vi "VsEP-Append Data.vi"(0 "path":path, 7 "Analysis":T2, 9 "Notes":string, 11 "error in (no error)":errorcluster) -> (15 "error out":errorcluster)   [LabVIEW 2020]
uses:
  Typedefs/VsEP-Analysis State.ctl
panel:
  in  "Data":T1
  out "path out":path
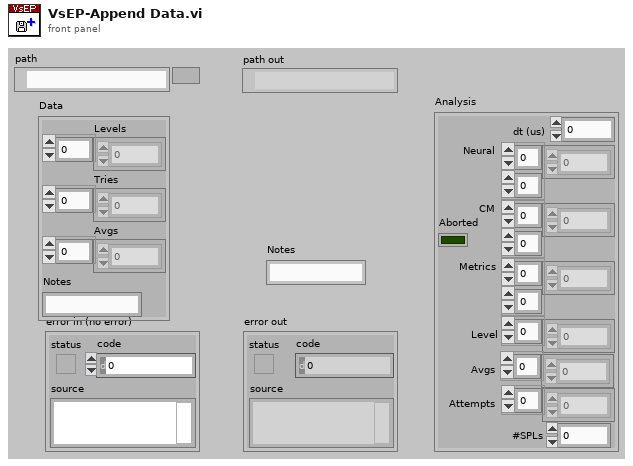
[diagram p1: front panel]
types:
  T1 = cluster{"Levels":dbl[], "Tries":i32[], "Avgs":i32[], "Notes":string}
  T2 = typedef "VsEP-Analysis State.ctl" = cluster{"dt (us)":dbl, "Neural":dbl[][], "CM":dbl[][], "Metrics":dbl[][], "Level":dbl[], "Avgs":i32[], "Attempts":i32[], "Aborted":bool, "#SPLs":i32}
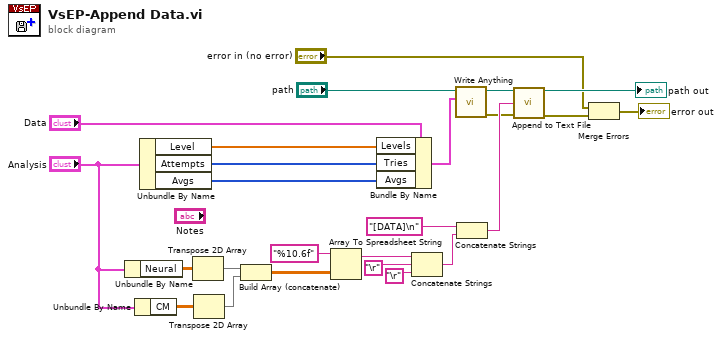
[diagram p0: block diagram]
diagram:
  n1 = Unbundle By Name("Analysis") -> ("Neural"=w15:dbl[][])
  n2 = Unbundle By Name("Analysis") -> ("CM"=w13:dbl[][])
  n3 = Unbundle By Name("Analysis") -> ("Level"=w9:dbl[], "Attempts"=w8:i32[], "Avgs"=w7:i32[])
  n4 = Transpose 2D Array(2D array=w15) -> (transposed array=w18:dbl[][])
  n5 = Transpose 2D Array(2D array=w13) -> (transposed array=w17:dbl[][])
  n6 = Build Array (concatenate)(w18, w17) -> (w16:dbl[][])
  n7 = Array To Spreadsheet String(array=w16, 3:"%10.6f") -> (spreadsheet string=w22:string)  [unwired: 1 in]
  n8 = Bundle By Name(cluster="Data", "Levels"=w9, "Tries"=w8, "Avgs"=w7) -> (w3:T1)
  n9 = Concatenate Strings(w22, "\r", "\r") -> (w2:string)
  n10 = call "Write Anything.vi"("Anything"=w3, "Path (dialog)"="path") -> ("Error Out"=w6:errorcluster, "Path out"=w5:path)  [unwired: 8 in]
  n11 = Concatenate Strings("[DATA]\n", w2) -> (w19:string)
  n12 = call "Append to Text File.vi"("file path"=w5, "text"=w19, "error in (no error)"=w6) -> ("file path out"=→"path out":path, "error out"=w24:errorcluster)  [unwired: 11 in]
  n13 = Merge Errors("error in (no error)", w24) -> (→"error out":errorcluster)
